vi "Start point.vi"(1 "Loop No":i32, 5 "Circuit cluster in":T1) -> (2 "Up circuit cluster out":T1, 13 "Down circuit cluster out":T1)   [LabVIEW 2016]
uses:
  TypeDefs/Circuit Cluster.ctl
  Classes/GateAbst/GateAbst.lvclass
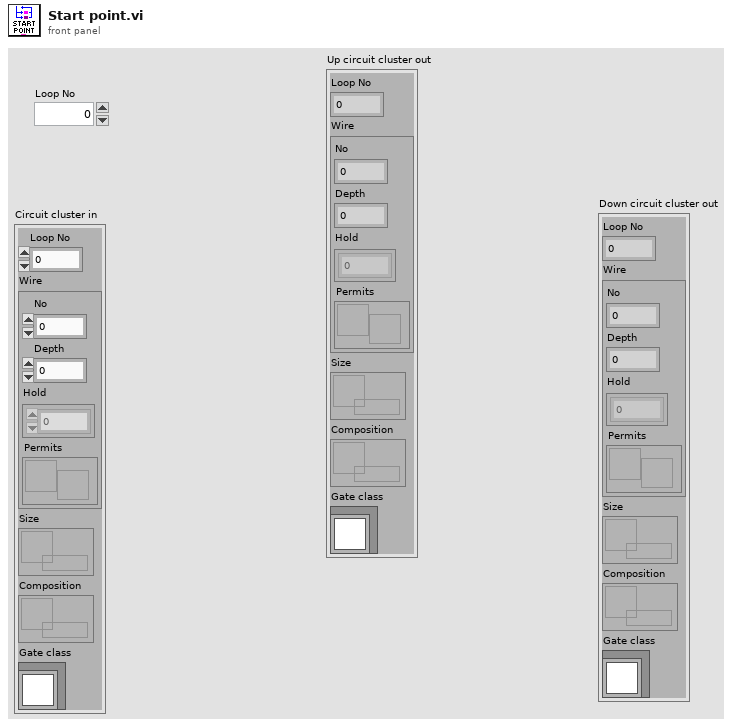
[diagram p1: front panel]
types:
  T1 = typedef "Circuit Cluster.ctl" = cluster{"Loop No":i32, "Wire":cluster{"No":i32, "Depth":i32, "Hold":i32[][], "Permits":refnum<notifier>}, "Size":refnum<queue>, "Composition":refnum<queue>, "Gate class":refnum<class "GateAbst.lvclass">}
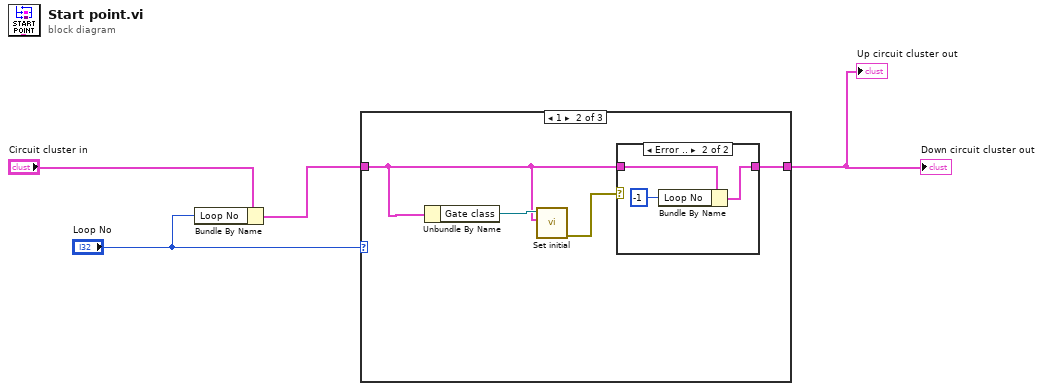
[diagram p0: block diagram]
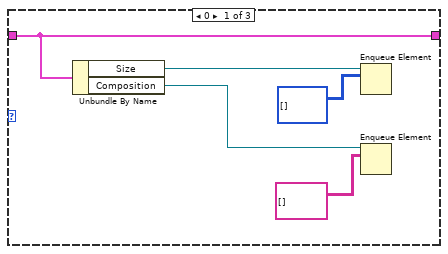
[diagram p2: hidden frame]
diagram:
  n1 = Bundle By Name(cluster="Circuit cluster in", "Loop No"="Loop No") -> (w2:T1)
  n2 = case shown="1" "Loop No" {
    tunnel: w2 -> [w7 w12 w18]
    tunnel: [w7 w11 w18] -> w4
    frame 0 {
      n3 = Unbundle By Name(w7) -> ("Size"=w6:refnum<queue>, "Composition"=w8:refnum<queue>)
      n4 = Enqueue Element(queue=w6, element=i32[][] []) -> ()  [unwired: 2 in, 3 out]
      n5 = Enqueue Element(queue=w8, element=string[][] []) -> ()  [unwired: 2 in, 3 out]
    }
    frame 1 {
      n6 = Unbundle By Name(w12) -> ("Gate class"=w13:refnum<class "GateAbst.lvclass">)
      n7 = call-dynamic "Set initial.vi"("Circuit cluster"=w12, "GateAbst in"=w13) -> ("error out"=w10:errorcluster)  [unwired: 8 in, 1 out]
      n8 = case shown="Error .." w10 {
        tunnel: w12 -> [w14 w17]
        tunnel: [w14 w16] -> w11
        frame No Error {
        }
        frame Error {
          n9 = Bundle By Name(cluster=w17, "Loop No"=-1) -> (w16:T1)
        }
      }
    }
    frame Default {
    }
  }
  "Down circuit cluster out" <- w4
  "Up circuit cluster out" <- w4
